vi "qn_armijo rule stepsize reduction.vi"(4 "s":dbl=1.0, 6 "F(X)":dbl, 7 "function and data":T1, 8 "error in (no error)":errorcluster, 9 "gradient":dbl[](array[numeric]), 10 "Direction":dbl[](array[numeric]), 11 "X":dbl[](array[numeric])) -> (0 "error out":errorcluster, 1 "number of function calls":i32, 2 "F(Xnew)":dbl, 3 "Xnew":dbl[](array[numeric]))   [LabVIEW 2017, in "NI_Gmath.lvlib"]
uses:
  <vilib>/gmath/NI_Gmath.lvlib
  <vilib>/gmath/NumericalOptimization/ucno_user function ref and data.ctl
  <vilib>/gmath/NumericalOptimization/ucno_user objective function ref.ctl
  <vilib>/Analysis/baseanly.llb/Real Dot Product.vi
  <vilib>/Analysis/NI_AALBase.lvlib
panel:
  in  "alpha":dbl=1.0
  in  "sigma":dbl=0.0001
  in  "beta":dbl=0.1
  # "`"
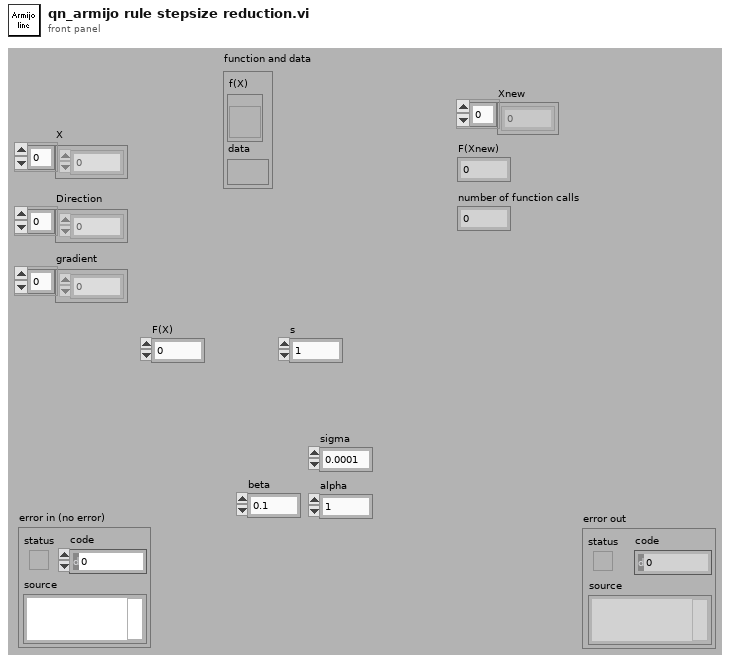
[diagram p1: front panel]
types:
  T1 = typedef "NI_Gmath.lvlib/ucno_user function ref and data.ctl" = cluster{"f(X)":T2, "data":variant}
  T2 = typedef "NI_Gmath.lvlib/ucno_user objective function ref.ctl" = refnum<vi>
  T3 = cluster{"objective function":bool, "gradient":bool}
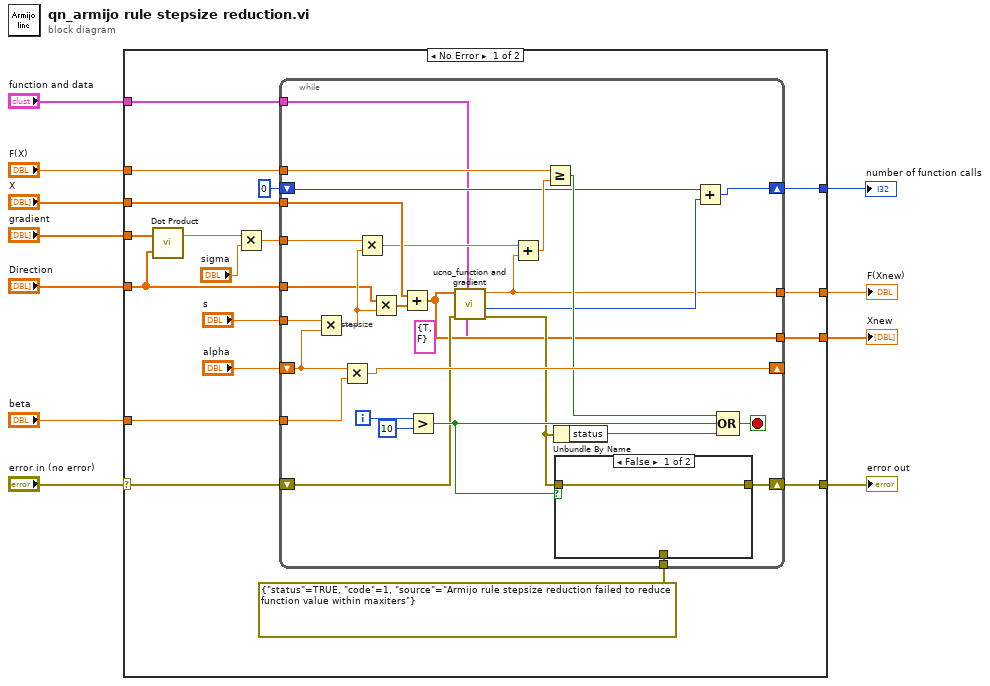
[diagram p0: block diagram]
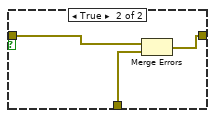
[diagram p2: hidden frame]
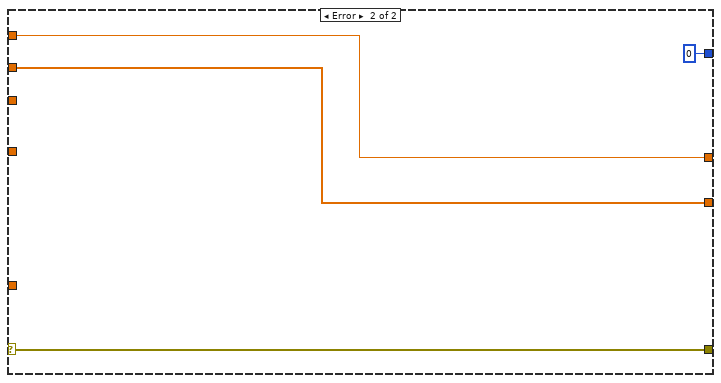
[diagram p3: hidden frame]
diagram:
  n1 = case shown="No Error" "error in (no error)" {
    selector: "error in (no error)" -> [w14 w64]
    tunnel: "gradient" -> [w29 _]
    tunnel: "Direction" -> [w28 _]
    tunnel: "X" -> [w27 w65]
    tunnel: "F(X)" -> [w26 w66]
    tunnel: "function and data" -> [w25 _]
    tunnel: "beta" -> [w20 _]
    tunnel: [w19 w66] -> w5
    tunnel: [w18 w65] -> w4
    tunnel: [w16 w64] -> w3
    tunnel: [w12 0] -> w1
    frame No Error {
      n2 = call-poly <vilib>:"Dot Product.vi"("Y Vector"=w28, "X Vector"=w29) -> ("X * Y"=w22:dbl)  [unwired: 1 out]
      n3 = Multiply(x=w22, y="sigma") -> (x*y=w21:dbl)
      n4 = while {
        shift-right: [w45] -> _
        shift-left: "alpha" -> [w46]
        tunnel: w28 -> [w57]
        tunnel: w27 -> [w56]
        tunnel: w26 -> [w54]
        tunnel: w21 -> [w51]
        tunnel: w25 -> [w33]
        tunnel: "s" -> [w48]
        tunnel: w20 -> [w47]
        tunnel: [w30] -> w19
        tunnel: [w34] -> w18
        shift-right: [w40] -> w16
        shift-left: w14 -> [w35]
        tunnel: errorcluster {"status"=TRUE, "code"=1, "source"="Armijo rule stepsize reduction failed to reduce function value within maxiters"} ("error in 2 (no error)") -> [w39]
        shift-right: [w38] -> w12
        shift-left: 0 -> [w37]
        i -> [w53]
        stop <- w49 stop-if-true
        # "stepsize"
        n5 = Multiply(x=w48, y=w46) -> (x*y=w58:dbl)
        n6 = Multiply(x=w46, y=w47) -> (x*y=w45:dbl)
        n7 = Multiply(x=w51, y=w58) -> (x*y=w43:dbl)
        n8 = Multiply(x=w57, y=w58) -> (x*y=w55:dbl[])
        n9 = Add(x=w56, y=w55) -> (x+y=w34:dbl[])
        n10 = Greater?(x=w53, y=10) -> (0:w41:bool)
        n11 = call <vilib>:"ucno_function and gradient.vi"("output control"=T3 {"objective function"=TRUE, "gradient"=FALSE}, "function and data"=w33, "error in (no error)"=w35, "X"=w34) -> ("error out"=w36:errorcluster, "number of function calls"=w31:i32, "f(X)"=w30:dbl)  [unwired: 4 in, 1 out]
        n12 = Add(x=w43, y=w30) -> (x+y=w50:dbl)
        n13 = Greater Or Equal?(x=w54, y=w50) -> (x >= y?=w44:bool)
        n14 = Unbundle By Name(w36) -> ("status"=w42:bool)
        n15 = case shown="False" w41 {
          tunnel: w36 -> [w59 w62]
          tunnel: [w59 w61] -> w40
          tunnel: w39 -> [_ w60]
          frame False {
          }
          frame True {
            n16 = Merge Errors(w62, w60) -> (w61:errorcluster)
          }
        }
        n17 = Add(x=w37, y=w31) -> (x+y=w38:i32)
        n18 = Compound Arithmetic op=OR(w44, w41, w42) -> (w49:bool)
      }
    }
    frame Error {
    }
  }
  "F(Xnew)" <- w5
  "Xnew" <- w4
  "error out" <- w3
  "number of function calls" <- w1
